vi "Begin.vi"(8 "error in":errorcluster) -> (0 "error out":errorcluster)   [LabVIEW 2016]
doc: "Called before other user functions, this VI is expected to open initial I/O refnums, load in file data, and do all program initialization. Notice that the <B>error out</B> terminal is simply used for data flow. Wiring it to other structures or subVIs ensures that this VI runs first."
uses:
  <vilib>/Rock Robotics/WPI/DriverStation/WPI_DriverStationRobotMode2.ctl
  <vilib>/Rock Robotics/WPI/Joystick/WPI_JoystickDeviceEnum.ctl
  <vilib>/Rock Robotics/SystemInterfaces/DIO/FPGA_DIOPWMChannel.ctl
  <vilib>/Rock Robotics/WPI/Solenoid/WPI_SolenoidChannel.ctl
  Robot Global Data.vi
  <vilib>/Rock Robotics/Network Tables/NT Write String Array.vi
  <vilib>/Rock Robotics/WPI/MotorControl/WPI_MotorControlOpen Talon.vi
  <vilib>/Rock Robotics/WPI/Utilities/WPI_GetSetVariantRefNum.vi
  <vilib>/Rock Robotics/WPI/Solenoid/WPI_SolenoidOpenSingle.vi
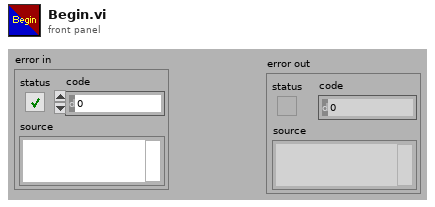
[diagram p1: front panel]
types:
  T1 = typedef "WPI_SolenoidChannel.ctl" = enum8{"Solenoid 0", "Solenoid 1", "Solenoid 2", "Solenoid 3", "Solenoid 4", "Solenoid 5", "Solenoid 6", "Solenoid 7", "Invalid"}
  T2 = typedef "FPGA_DIOPWMChannel.ctl" = enum8{"PWM 0", "PWM 1", "PWM 2", "PWM 3", "PWM 4", "PWM 5", "PWM 6", "PWM 7", "PWM 8", "PWM 9", "PWM MXP 0", "PWM MXP 1", "PWM MXP 2", "PWM MXP 3", "PWM MXP 4", "PWM MXP 5", "PWM MXP 6", "PWM MXP 7", "PWM MXP 8", "PWM MXP 9", "Invalid"}
  T3 = typedef "WPI_JoystickDeviceEnum.ctl" = enum16{"USB 0", "USB 1", "USB 2", "USB 3", "USB 4", "USB 5"}
  T4 = typedef "WPI_DriverStationRobotMode2.ctl" = enum16{"Autonomous Disabled", "Autonomous Enabled", "Teleop Disabled", "Teleop Enabled", "Disconnected", "Finish", "Test Disabled", "Test Enabled", "Emergency Stopped"}
  T5 = typedef "WPI_CompressorDevRef.ctl" = cluster{"DevStatus":errorcluster, "Pneumatics Control Module":u8}
  T6 = typedef "WPI_JoystickDevRef.ctl" = cluster{"Device":T3}
  T7 = typedef "WPI_MotorControlDeviceRef.ctl" = cluster{"DeviceStatus":errorcluster, "Type":T8, "PWM":cluster{"PWM Channel":T2, "DeadBand":T9}, "CAN":cluster{"Device Number":u8, "SetOutput VI Ref":variant, "GetOutput VI Ref":variant, "Enable VI Ref":variant, "Disable VI Ref":variant, "Data":variant}, "Invert":bool}
  T8 = typedef "WPI_MotorControlType.ctl" = enum16{"PWM", "CAN"}
  T9 = typedef "WPI_PWMDeadband.ctl" = cluster{"Name":string, "maxPositivePwm":i32, "minPositivePwm":i32, "centerPwm":i32, "maxNegativePwm":i32, "minNegativePwm":i32, "angularRange":u16}
  T10 = typedef "WPI_SolenoidDevRef.ctl" = cluster{"DevStatus":errorcluster, "Pneumatics Control Module":u8, "Forward Solenoid Channel":T1, "Reverse Solenoid Channel":T1}
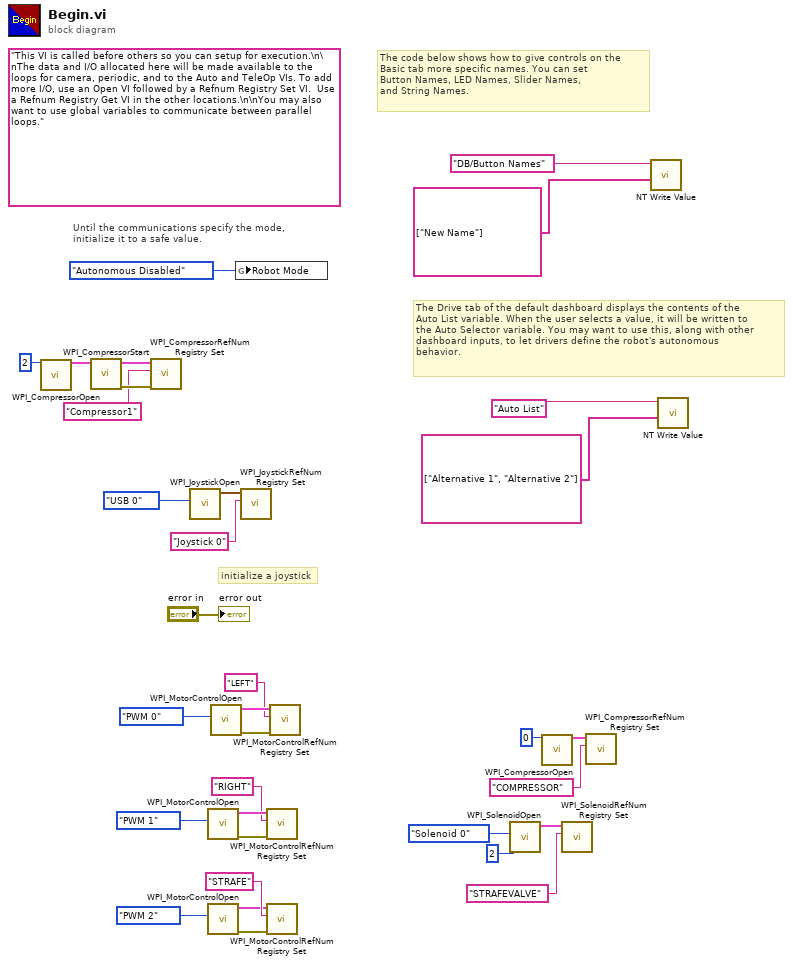
[diagram p0: block diagram]
diagram:
  (unwired) "This VI is called before others so you can setup for execution.\n\nThe data and I/O allocated here will be made available to the loops for camera, periodic, and to the Auto and TeleOp VIs. To add more I/O, use an Open VI followed by a Refnum Registry Set VI.  Use a Refnum Registry Get VI in the other locations.\n\nYou may also want to use global variables to communicate between parallel loops."
  # "The Drive tab of the default dashboard displays the contents of the\nAuto List variable. When the user selects a value, it will be written to\nthe Auto Selector variable. You may want to use this, along with other\ndashboard inputs, to let drivers define the robot's autonomous\nbehavior."
  # "The code below shows how to give controls on the\nBasic tab more specific names. You can set\nButton Names, LED Names, Slider Names,\nand String Names."
  # "initialize a joystick"
  # "Until the communications specify the mode,\ninitialize it to a safe value."
  n1 = call <vilib>:"WPI_CompressorOpen.vi"("Pneumatics Control Module (0)"=u8 2) -> ("CompressorDevRef"=w6:T5)  [unwired: 13 in, 1 out]
  n2 = call <vilib>:"WPI_CompressorStart.vi"("CompressorDevRef"=w6) -> ("error out"=w4:errorcluster, "CompressorDevRef"=w3:T5)  [unwired: 2 in, 7 out]
  n3 = call <vilib>:"WPI_CompressorRefNum Registry Set.vi"("error in (no error)"=w4, "refnum name"="Compressor1", "CompressorDevRef"=w3) -> ()  [unwired: 7 in, 2 out]
  n4 = call <vilib>:"WPI_JoystickOpen.vi"("JoystickDevice"=WPI_JoystickDeviceEnum."USB 0") -> ("JoystickDevRef"=w31:T6)  [unwired: 10 in]
  n5 = call-poly <vilib>:"WPI_MotorControlOpen.vi"("PWM Channel"=FPGA_DIOPWMChannel."PWM 1") -> ("error out"=w15:errorcluster, "MotorControlDeviceRef"=w14:T7)  [unwired: 9 in]
  n6 = call-poly <vilib>:"WPI_MotorControlOpen.vi"("PWM Channel"=FPGA_DIOPWMChannel."PWM 2") -> ("error out"=w22:errorcluster, "MotorControlDeviceRef"=w21:T7)  [unwired: 9 in]
  n7 = call-poly <vilib>:"WPI_MotorControlOpen.vi"("PWM Channel"=FPGA_DIOPWMChannel."PWM 0") -> ("error out"=w19:errorcluster, "MotorControlDeviceRef"=w18:T7)  [unwired: 9 in]
  n8 = global write "Robot Global Data.vi" "Robot Mode"(WPI_DriverStationRobotMode2."Autonomous Disabled" ("Robot Mode")) -> ()
  n9 = call <vilib>:"WPI_JoystickRefNum Registry Set.vi"("refnum name"="Joystick 0", "JoystickDevRef"=w31) -> ()  [unwired: 8 in, 2 out]
  n10 = call <vilib>:"WPI_MotorControlRefNum Registry Set.vi"("error in (no error)"=w15, "refnum name"="RIGHT", "MotorControlDevRef"=w14) -> ()  [unwired: 7 in, 2 out]
  n11 = call <vilib>:"WPI_MotorControlRefNum Registry Set.vi"("error in (no error)"=w22, "refnum name"="STRAFE", "MotorControlDevRef"=w21) -> ()  [unwired: 7 in, 2 out]
  n12 = call <vilib>:"WPI_MotorControlRefNum Registry Set.vi"("error in (no error)"=w19, "refnum name"="LEFT", "MotorControlDevRef"=w18) -> ()  [unwired: 7 in, 2 out]
  n13 = call-poly <vilib>:"WPI_SolenoidOpen.vi"("Solenoid Channel"=WPI_SolenoidChannel."Solenoid 0", "Pneumatics Control Module (0)"=u8 2) -> ("SolenoidDevRef"=w11:T10)  [unwired: 8 in, 1 out]
  n14 = call <vilib>:"WPI_CompressorOpen.vi"("Pneumatics Control Module (0)"=u8 0) -> ("CompressorDevRef"=w9:T5)  [unwired: 13 in, 1 out]
  n15 = call <vilib>:"WPI_SolenoidRefNum Registry Set.vi"("refnum name"="STRAFEVALVE", "SolenoidDevRef"=w11) -> ()  [unwired: 8 in, 2 out]
  n16 = call <vilib>:"WPI_CompressorRefNum Registry Set.vi"("refnum name"="COMPRESSOR", "CompressorDevRef"=w9) -> ()  [unwired: 8 in, 2 out]
  n17 = call-poly <vilib>:"NT Write Value.vi"("String Array"=string[] ["New Name"], "Name"="DB/Button Names") -> ()  [unwired: 9 in, 1 out]
  n18 = call-poly <vilib>:"NT Write Value.vi"("String Array"=string[] ["Alternative 1", "Alternative 2"], "Name"="Auto List") -> ()  [unwired: 9 in, 1 out]
  "error out" <- "error in"
